vi "QA.vi"(8 "ERRIN":errorcluster caption="entrée d'erreur (pas d'erreur)") -> (0 "ERROUT":errorcluster caption="sortie d'erreur", 3 "DATA OUT":string)   [LabVIEW 2020]
uses:
  <vilib>/Instr/_visa.llb/VISA Configure Serial Port (Instr).vi
panel:
  # "<\\B20\\BE:(A\\CC\\A9:P\\D2\\C5SS\\C9\\CFN\\A0HAU\\D4\\C5\\8D\\n"
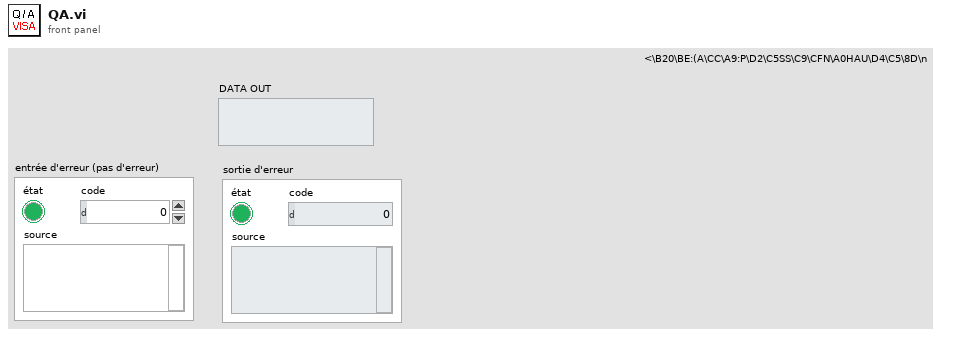
[diagram p1: front panel]
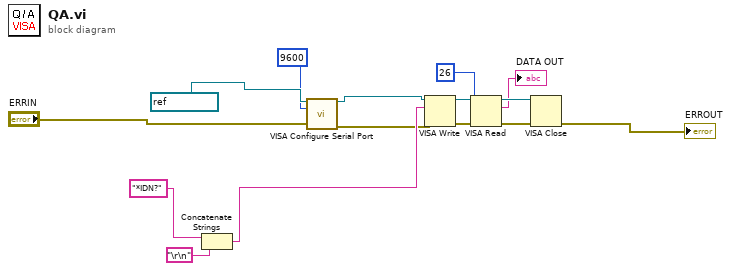
[diagram p0: block diagram]
diagram:
  n1 = Concatenate Strings("*IDN?" ("buffer d'écriture"), "\r\n") -> (w12:string)
  n2 = call-poly "VISA Configure Serial Port"("VISA resource name"=refnum<visa-resource-name> "COM10" ("Refnum VISA en sortie"), "baud rate (9600)"=u32 9600, "error in (no error)"="ERRIN") -> ("VISA resource name out"=w2:refnum<visa-resource-name>, "error out"=w3:errorcluster)  [unwired: 11 in]
  n3 = VISA Write(VISA resource name=w2, write buffer=w12, error in (no error)=w3) -> (VISA resource name out=w4:refnum<visa-resource-name>, error out=w7:errorcluster)  [unwired: 1 out]
  n4 = VISA Read(VISA resource name=w4, byte count=u32 26 ("nombre d'octets"), error in (no error)=w7) -> (VISA resource name out=w8:refnum<visa-resource-name>, read buffer=→"DATA OUT":string, error out=w9:errorcluster)  [unwired: 1 out]
  n5 = VISA Close(VISA resource name=w8, error in (no error)=w9) -> (error out=→"ERROUT":errorcluster)
